vi "Format Refs to Engine.vi"(10 "Output References":T1 {"Holding Registers" format="%.0x"; "Input Registers" format="%.0x"; "Discrete Inputs" format="%.0x"; "Coils" format="%.0x"}, 11 "Input References":T1 {"Holding Registers" format="%.0x"; "Input Registers" format="%.0x"; "Discrete Inputs" format="%.0x"; "Coils" format="%.0x"}) -> (3 "Refs out":T3(array[cluster]) {"VS Refs" format="%.0x"})   [LabVIEW 2015]
uses:
  <vilib>/NI Veristand/Custom Device API/Custom Device Item Ref.ctl
  Shared/Controls/Data Model/References.ctl
  Shared/Constants.vi
  <vilib>/NI VeriStand/Custom Device API/Custom Device API.lvlib
  Shared/Modbus Master Shared.lvlib
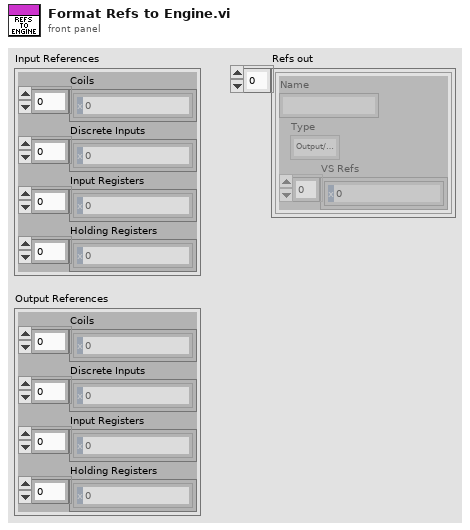
[diagram p1: front panel]
types:
  T1 = typedef "Modbus Master Shared.lvlib/References.ctl" = cluster{"Coils":T2[], "Discrete Inputs":T2[], "Input Registers":T2[], "Holding Registers":T2[]}
  T2 = typedef "Custom Device API.lvlib/Custom Device Item Ref.ctl" = u64
  T3 = cluster{"Name":string, "Type":enum16{"Output/Write", "Input/Read", "Input/ReadWrite"}, "VS Refs":T2[]}[]
  T4 = enum16{"Output/Write", "Input/Read", "Input/ReadWrite"}
  T5 = cluster{"Name":string, "Type":enum16{"Output/Write", "Input/Read", "Input/ReadWrite"}, "VS Refs":T2[]}
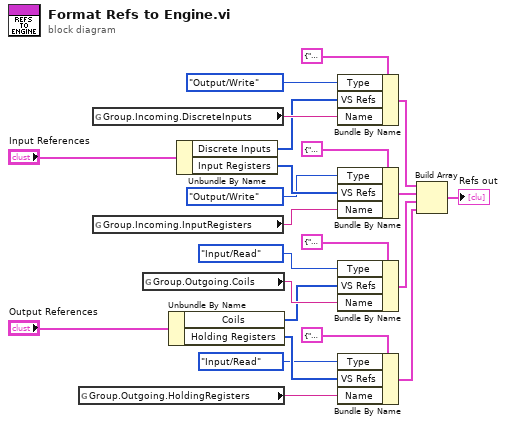
[diagram p0: block diagram]
diagram:
  n1 = global read "Constants.vi" "Group.Outgoing.HoldingRegisters"() -> (w1:string)
  n2 = global read "Constants.vi" "Group.Incoming.DiscreteInputs"() -> (w21:string)
  n3 = global read "Constants.vi" "Group.Incoming.InputRegisters"() -> (w22:string)
  n4 = global read "Constants.vi" "Group.Outgoing.Coils"() -> (w23:string)
  n5 = Unbundle By Name("Output References") -> ("Coils"=w12:T2[], "Holding Registers"=w13:T2[])
  n6 = Unbundle By Name("Input References") -> ("Discrete Inputs"=w19:T2[], "Input Registers"=w20:T2[])
  n7 = Bundle By Name(cluster=T5 {"Name"="", "Type"=enum."Output/Write", "VS Refs"=[]} ("Group"), "Type"=T4."Output/Write", "VS Refs"=w19, "Name"=w21) -> (w14:T5)
  n8 = Bundle By Name(cluster=T5 {"Name"="", "Type"=enum."Output/Write", "VS Refs"=[]} ("Group"), "Type"=T4."Output/Write", "VS Refs"=w20, "Name"=w22) -> (w15:T5)
  n9 = Bundle By Name(cluster=T5 {"Name"="", "Type"=enum."Output/Write", "VS Refs"=[]} ("Group"), "Type"=T4."Input/Read", "VS Refs"=w12, "Name"=w23) -> (w16:T5)
  n10 = Bundle By Name(cluster=T5 {"Name"="", "Type"=enum."Output/Write", "VS Refs"=[]} ("Group"), "Type"=T4."Input/Read", "VS Refs"=w13, "Name"=w1) -> (w17:T5)
  n11 = Build Array(w14, w15, w16, w17) -> (→"Refs out":T3)
